vi "Main.vi"() -> ()   [LabVIEW 2018] (continued)
              tunnel: w2112 -> [w2128 w2142]
              tunnel: w2115 -> [w2127 w2155]
              tunnel: w2114 -> [w2126 w2154]
              frame False {
                n1936 = call "SQL_Update.vi"("查询语句"=w2128, "表名"="Online", "error in (no error)"=w2126, "列名对应的值"=w2135, "列名"=string[] ["Last_Station", "Last_Result", "ST403_Date", "ST403_Time", "ST403_Package_Result", "ST403_Circlip_5026621", "ST403_Jump_Ring_Data", "ST403_Jump_Ring_Tolerance", "ST402_Camera_Shield"], "connection reference"=w2127) -> ("error out"=w2130:errorcluster)  [unwired: 4 in, 1 out]
                n1937 = Unbundle By Name(w2130) -> ("status"=w2134:bool)
                n1938 = Equal?(x=w2129, y="") -> (x = y?=w2132:bool)
                n1939 = Or(x=w2134, y=w2132) -> (x .or. y?=w2131:bool)
                n1940 = case shown="假" w2131 {
                  tunnel: ["1" ("数据保存请求回复") "2" ("数据保存请求回复")] -> w2136
                  frame False {
                  }
                  frame True {
                  }
                }
              }
              frame True {
                w2150 = 0 ("索引 (行)")
                n1941 = call "SQL_Select.vi"("要读取的列名"=string[] ["[403]"], "表名"="Rework_List", "error in (no error)"=w2154, "查询语句"=w2142, "查询条件"=TRUE, "connection reference"=w2155) -> ("error out"=w2145:errorcluster, "数据"=w2151:string[][], "connection reference out"=w2146:T12)  [unwired: 3 in]
                n1942 = Index Array(array=w2151, index (row)=w2150, index (col)=w2150) -> (element=w2149:string)
                n1943 = Equal?(x=w2149, y="T") -> (x = y?=w2147:bool)
                n1944 = case shown="真" w2147 {
                  tunnel: w2146 -> [w2163 w2182]
                  tunnel: w2145 -> [w2164 w2181]
                  tunnel: w2144 -> [w2162 w2188]
                  tunnel: w2143 -> [w2159 w2183]
                  tunnel: w2142 -> [w2161 w2173]
                  tunnel: [w2158 w2175] -> w2141
                  tunnel: [w2160 w2174] -> w2140
                  frame False {
                    n1945 = call "SQL_Update.vi"("查询语句"=w2161, "表名"="Online", "error in (no error)"=w2164, "列名对应的值"=w2162, "列名"=string[] ["Last_Station", "Last_Result", "ST403_Date", "ST403_Time", "ST403_Package_Result", "ST403_Circlip_5026621", "ST403_Jump_Ring_Data", "ST403_Jump_Ring_Tolerance", "ST402_Camera_Shield"], "connection reference"=w2163) -> ("error out"=w2160:errorcluster)  [unwired: 4 in, 1 out]
                    n1946 = Unbundle By Name(w2160) -> ("status"=w2168:bool)
                    n1947 = Equal?(x=w2159, y="") -> (x = y?=w2166:bool)
                    n1948 = Or(x=w2168, y=w2166) -> (x .or. y?=w2165:bool)
                    n1949 = case shown="假" w2165 {
                      tunnel: ["1" ("数据保存请求回复") "2" ("数据保存请求回复")] -> w2158
                      frame False {
                      }
                      frame True {
                      }
                    }
                  }
                  frame True {
                    n1950 = Delete From Array(array=w2188, length=2 ("长度"), index=0 ("索引")) -> (deleted portion=w2176:string[], array with subset deleted=w2185:string[])
                    n1951 = call "SQL_Update.vi"("查询语句"=w2173, "表名"="Online", "error in (no error)"=w2181, "列名对应的值"=w2176, "列名"=string[] ["Last_Station", "Last_Result"], "connection reference"=w2182) -> ("error out"=w2180:errorcluster, "connection reference 2"=w2179:T12)  [unwired: 4 in]
                    n1952 = call "SQL_Update.vi"("查询语句"=w2173, "表名"="Rework", "error in (no error)"=w2180, "列名对应的值"=w2185, "列名"=string[] ["ST403_Date", "ST403_Time", "ST403_Package_Result", "ST403_Circlip_5026621", "ST403_Jump_Ring_Data", "ST403_Jump_Ring_Tolerance", "ST402_Camera_Shield"], "connection reference"=w2179) -> ("error out"=w2174:errorcluster)  [unwired: 4 in, 1 out]
                    n1953 = Unbundle By Name(w2174) -> ("status"=w2191:bool)
                    n1954 = Equal?(x="", y=w2183) -> (x = y?=w2190:bool)
                    n1955 = Or(x=w2191, y=w2190) -> (x .or. y?=w2189:bool)
                    n1956 = case shown="真" w2189 {
                      tunnel: ["1" ("数据保存请求回复") "2" ("数据保存请求回复")] -> w2175
                      frame False {
                      }
                      frame True {
                      }
                    }
                  }
                }
              }
            }
            n1957 = Delete From Array(array=w2088, length=2 ("长度"), index=0 ("索引")) -> (array with subset deleted=w2120:string[])  [unwired: 1 out]
            n1958 = Insert Into Array(array=string[] [] ("数组"), index=0 ("索引"), new element=w2113) -> (w2123:string[])
            n1959 = Insert Into Array(array=w2120, index=2 ("索引"), new element=w2092) -> (w2119:string[])
            n1960 = Bundle By Name(cluster=cluster{"Data":string[], "State":T1} {"Data"=[], "State"=enum."PLC通讯初始化"} ("元素"), "Data"=w2123, "State"=状态2."数据保存回复3") -> (w2122:cluster{"Data":string[], "State":T1})
            n1961 = Insert Into Array(array=string[][] [] ("数组"), index (row)=0 ("索引 (行)"), new element=w2119) -> (w2121:string[][])  [unwired: 1 in]
            n1962 = Enqueue Element(queue=w2093, element=w2122) -> ()  [unwired: 2 in, 3 out]
            n1963 = Transpose 2D Array(2D array=w2121) -> (transposed array=w2091:string[][])
            n1964 = property on="ST40-3_DATA" class="MCListbox (严格)"("ItemNames"=w2091) -> ()  [unwired: 2 in, 2 out]
            "ST403数据读取（事件）" <- FALSE ("ST403数据读取（事件）")
          }
          event "ST502扫码请求(事件)": Value Change {
            n1965 = event-data() -> ()  [unwired: 1 in, 1 out]
            n1966 = local read "502二维码"() -> (w2195:string)
            n1967 = Concatenate Strings("Where QRCode='" ("查询语句"), w2195, "'" ("字符串")) -> (w2221:string)
            n1968 = call "SQL_Select.vi"("要读取的列名"=string[] ["Last_Station", "Last_Result"], "表名"="Online", "error in (no error)"=w2200, "查询语句"=w2221, "查询条件"=TRUE, "connection reference"=w2201) -> ("error out"=w2198:errorcluster, "数据"=w2220:string[][])  [unwired: 3 in, 1 out]
            n1969 = case shown="无错误" w2198 {
              tunnel: w2220 -> [w2234 _]
              tunnel: ["1" ("右扫码请求回复") "2" ("右扫码请求回复")] -> w2213
              tunnel: [w2229 w2235] -> w2212
              tunnel: [w2228 w2235] -> w2211
              frame No Error {
                n1970 = Index Array(array=w2234, index (row)=0 ("索引 (行)")) -> (element=w2231:string[])  [unwired: 1 in]
                n1971 = Index Array(array=w2231, index #1=0 ("索引 (行)")) -> (element #1=w2229:string, element #2=w2228:string)  [unwired: 1 in]
                "上一站号 (502)" <- w2229
                "上一站结果 (502)" <- w2228
              }
              frame Error {
                w2235 = ""
              }
            }
            n1972 = Insert Into Array(array=string[] [] ("数组"), index=0 ("索引"), new element #1=w2213, new element #2=w2212, new element #3=w2211) -> (w2217:string[])
            n1973 = Format Date/Time String(time format string (%c)="%Y-%m-%d" ("时间格式字符串(%c)")) -> (date/time string=w2209:string)  [unwired: 2 in]
            n1974 = Get Date/Time String() -> (time string=w2208:string)  [unwired: 3 in, 1 out]
            n1975 = Bundle By Name(cluster=cluster{"Data":string[], "State":T1} {"Data"=[], "State"=enum."PLC通讯初始化"} ("元素"), "Data"=w2217, "State"=状态2."扫码回复") -> (w2218:cluster{"Data":string[], "State":T1})
            n1976 = Insert Into Array(array=string[] [] ("数组"), index=0 ("索引"), new element #1=w2209, new element #2=w2208, new element #3=w2195) -> (w2205:string[])
            n1977 = Enqueue Element(queue=w2199, element=w2218) -> ()  [unwired: 2 in, 3 out]
            n1978 = Insert Into Array(array=string[][] [] ("数组"), index (row)=0 ("索引 (行)"), new element=w2205) -> (w2202:string[][])  [unwired: 1 in]
            n1979 = Transpose 2D Array(2D array=w2202) -> (transposed array=w2196:string[][])
            n1980 = property on="ST50-2_DATA" class="MCListbox (严格)"("ItemNames"=w2196) -> ()  [unwired: 2 in, 2 out]
            "ST502扫码请求(事件)" <- FALSE ("ST50扫码请求(事件)")
          }
          event "ST502数据读取（事件）": Value Change {
            w2249 = 0 ("索引 (行)")
            n1981 = event-data() -> ()  [unwired: 1 in, 1 out]
            n1982 = local read "502二维码"() -> (w2237:string)
            n1983 = Dequeue Element(queue=w2260, timeout in ms (-1)=10 ("超时毫秒(-1)")) -> (element=w2241:string[])  [unwired: 1 in, 3 out]
            n1984 = Concatenate Strings("Where QRCode='" ("查询语句"), w2237, "'" ("字符串")) -> (w2251:string)
            n1985 = call "SQL_Select.vi"("要读取的列名"=string[] ["Rework_Status"], "表名"="Online", "error in (no error)"=w2243, "查询语句"=w2251, "查询条件"=TRUE, "connection reference"=w2242) -> ("error out"=w2244:errorcluster, "数据"=w2250:string[][], "connection reference out"=w2245:T12)  [unwired: 3 in]
            n1986 = Index Array(array=w2250, index (row)=w2249, index (col)=w2249) -> (element=w2248:string)
            n1987 = Equal?(x=w2248, y="T") -> (x = y?=w2246:bool)
            n1988 = case shown="真" w2246 {
              tunnel: [w2287 w2292] -> w2240
              tunnel: w2241 -> [w2286 w2295]
              tunnel: [w2281 w2291] -> w2239
              tunnel: w2237 -> [w2280 w2294]
              tunnel: w2251 -> [w2279 w2293]
              tunnel: w2245 -> [w2278 w2306]
              tunnel: w2244 -> [w2277 w2305]
              frame False {
                n1989 = call "SQL_Update.vi"("查询语句"=w2279, "表名"="Online", "error in (no error)"=w2277, "列名对应的值"=w2286, "列名"=string[] ["Last_Station", "Last_Result", "ST502_Date", "ST502_Time", "ST502_Package_Result", "ST502_Form_Seal_5026860", "ST502_Support_Ring_5027083", "ST502_O_Ring_M0104976", "ST502_Pressure_Plate_M0105053", "ST502_Camera_Shield", "ST502_Seal_Ring_TestValue", "ST502_Seal_Ring_SetValue"], "connection reference"=w2278) -> ("error out"=w2281:errorcluster)  [unwired: 4 in, 1 out]
                n1990 = Unbundle By Name(w2281) -> ("status"=w2285:bool)
                n1991 = Equal?(x=w2280, y="") -> (x = y?=w2283:bool)
                n1992 = Or(x=w2285, y=w2283) -> (x .or. y?=w2282:bool)
                n1993 = case shown="假" w2282 {
                  tunnel: ["1" ("数据保存请求回复") "2" ("数据保存请求回复")] -> w2287
                  frame False {
                  }
                  frame True {
                  }
                }
              }
              frame True {
                w2301 = 0 ("索引 (行)")
                n1994 = call "SQL_Select.vi"("要读取的列名"=string[] ["[502]"], "表名"="Rework_List", "error in (no error)"=w2305, "查询语句"=w2293, "查询条件"=TRUE, "connection reference"=w2306) -> ("error out"=w2296:errorcluster, "数据"=w2302:string[][], "connection reference out"=w2297:T12)  [unwired: 3 in]
                n1995 = Index Array(array=w2302, index (row)=w2301, index (col)=w2301) -> (element=w2300:string)
                n1996 = Equal?(x=w2300, y="T") -> (x = y?=w2298:bool)
                n1997 = case shown="假" w2298 {
                  tunnel: w2297 -> [w2314 w2333]
                  tunnel: w2296 -> [w2315 w2332]
                  tunnel: w2295 -> [w2313 w2339]
                  tunnel: w2294 -> [w2310 w2334]
                  tunnel: w2293 -> [w2312 w2324]
                  tunnel: [w2309 w2326] -> w2292
                  tunnel: [w2311 w2325] -> w2291
                  frame False {
                    n1998 = call "SQL_Update.vi"("查询语句"=w2312, "表名"="Online", "error in (no error)"=w2315, "列名对应的值"=w2313, "列名"=string[] ["Last_Station", "Last_Result", "ST502_Date", "ST502_Time", "ST502_Package_Result", "ST502_Form_Seal_5026860", "ST502_Support_Ring_5027083", "ST502_O_Ring_M0104976", "ST502_Pressure_Plate_M0105053", "ST502_Camera_Shield", "ST502_Seal_Ring_TestValue", "ST502_Seal_Ring_SetValue"], "connection reference"=w2314) -> ("error out"=w2311:errorcluster)  [unwired: 4 in, 1 out]
                    n1999 = Unbundle By Name(w2311) -> ("status"=w2319:bool)
                    n2000 = Equal?(x=w2310, y="") -> (x = y?=w2317:bool)
                    n2001 = Or(x=w2319, y=w2317) -> (x .or. y?=w2316:bool)
                    n2002 = case shown="假" w2316 {
                      tunnel: ["1" ("数据保存请求回复") "2" ("数据保存请求回复")] -> w2309
                      frame False {
                      }
                      frame True {
                      }
                    }
                  }
                  frame True {
                    n2003 = Delete From Array(array=w2339, length=2 ("长度"), index=0 ("索引")) -> (deleted portion=w2327:string[], array with subset deleted=w2336:string[])
                    n2004 = call "SQL_Update.vi"("查询语句"=w2324, "表名"="Online", "error in (no error)"=w2332, "列名对应的值"=w2327, "列名"=string[] ["Last_Station", "Last_Result"], "connection reference"=w2333) -> ("error out"=w2331:errorcluster, "connection reference 2"=w2330:T12)  [unwired: 4 in]
                    n2005 = call "SQL_Update.vi"("查询语句"=w2324, "表名"="Rework", "error in (no error)"=w2331, "列名对应的值"=w2336, "列名"=string[] ["ST502_Date", "ST502_Time", "ST502_Package_Result", "ST502_Form_Seal_5026860", "ST502_Support_Ring_5027083", "ST502_O_Ring_M0104976", "ST502_Pressure_Plate_M0105053", "ST502_Camera_Shield", "ST502_Seal_Ring_TestValue", "ST502_Seal_Ring_SetValue"], "connection reference"=w2330) -> ("error out"=w2325:errorcluster)  [unwired: 4 in, 1 out]
                    n2006 = Unbundle By Name(w2325) -> ("status"=w2342:bool)
                    n2007 = Equal?(x="", y=w2334) -> (x = y?=w2341:bool)
                    n2008 = Or(x=w2342, y=w2341) -> (x .or. y?=w2340:bool)
                    n2009 = case shown="真" w2340 {
                      tunnel: ["1" ("数据保存请求回复") "2" ("数据保存请求回复")] -> w2326
                      frame False {
                      }
                      frame True {
                      }
                    }
                  }
                }
              }
            }
            n2010 = Delete From Array(array=w2241, length=2 ("长度"), index=0 ("索引")) -> (array with subset deleted=w2263:string[])  [unwired: 1 out]
            n2011 = Insert Into Array(array=w2263, index=2 ("索引"), new element=w2237) -> (w2261:string[])
            n2012 = Insert Into Array(array=string[] [] ("数组"), index=0 ("索引"), new element=w2240) -> (w2273:string[])
            n2013 = Bundle By Name(cluster=cluster{"Data":string[], "State":T1} {"Data"=[], "State"=enum."PLC通讯初始化"} ("元素"), "Data"=w2273, "State"=状态2."数据保存回复") -> (w2269:cluster{"Data":string[], "State":T1})
            n2014 = Insert Into Array(array=string[][] [] ("数组"), index (row)=0 ("索引 (行)"), new element=w2261) -> (w2266:string[][])  [unwired: 1 in]
            n2015 = Transpose 2D Array(2D array=w2266) -> (transposed array=w2238:string[][])
            n2016 = Enqueue Element(queue=w2259, element=w2269) -> ()  [unwired: 2 in, 3 out]
            n2017 = property on="ST50-2_DATA" class="MCListbox (严格)"("ItemNames"=w2238) -> ()  [unwired: 2 in, 2 out]
            "ST502数据读取（事件）" <- FALSE ("ST50数据读取（事件）")
          }
          event "ST503扫码请求(事件)": Value Change {
            n2018 = event-data() -> ()  [unwired: 1 in, 1 out]
            n2019 = local read "503二维码"() -> (w2346:string)
            n2020 = Concatenate Strings("Where QRCode='" ("查询语句"), w2346, "'" ("字符串")) -> (w2350:string)
            n2021 = call "SQL_Select.vi"("要读取的列名"=string[] ["Last_Station", "Last_Result"], "表名"="Online", "error in (no error)"=w2348, "查询语句"=w2350, "查询条件"=TRUE, "connection reference"=w2349) -> ("error out"=w2352:errorcluster, "数据"=w2372:string[][])  [unwired: 3 in, 1 out]
            n2022 = case shown="无错误" w2352 {
              tunnel: w2372 -> [w2385 _]
              tunnel: ["1" ("右扫码请求回复") "2" ("右扫码请求回复")] -> w2365
              tunnel: [w2380 w2386] -> w2364
              tunnel: [w2379 w2386] -> w2363
              frame No Error {
                n2023 = Index Array(array=w2385, index (row)=0 ("索引 (行)")) -> (element=w2382:string[])  [unwired: 1 in]
                n2024 = Index Array(array=w2382, index #1=0 ("索引 (行)")) -> (element #1=w2380:string, element #2=w2379:string)  [unwired: 1 in]
                "上一站号 (503)" <- w2380
                "上一站结果 (503)" <- w2379
              }
              frame Error {
                w2386 = ""
              }
            }
            n2025 = Insert Into Array(array=string[] [] ("数组"), index=0 ("索引"), new element #1=w2365, new element #2=w2364, new element #3=w2363) -> (w2369:string[])
            n2026 = Format Date/Time String(time format string (%c)="%Y-%m-%d" ("时间格式字符串(%c)")) -> (date/time string=w2361:string)  [unwired: 2 in]
            n2027 = Get Date/Time String() -> (time string=w2360:string)  [unwired: 3 in, 1 out]
            n2028 = Bundle By Name(cluster=cluster{"Data":string[], "State":T1} {"Data"=[], "State"=enum."PLC通讯初始化"} ("元素"), "Data"=w2369, "State"=状态2."扫码回复2") -> (w2370:cluster{"Data":string[], "State":T1})
            n2029 = Insert Into Array(array=string[] [] ("数组"), index=0 ("索引"), new element #1=w2361, new element #2=w2360, new element #3=w2346) -> (w2357:string[])
            n2030 = Enqueue Element(queue=w2353, element=w2370) -> ()  [unwired: 2 in, 3 out]
            n2031 = Insert Into Array(array=string[][] [] ("数组"), index (row)=0 ("索引 (行)"), new element=w2357) -> (w2354:string[][])  [unwired: 1 in]
            n2032 = Transpose 2D Array(2D array=w2354) -> (transposed array=w2347:string[][])
            n2033 = property on="ST50-3_DATA" class="MCListbox (严格)"("ItemNames"=w2347) -> ()  [unwired: 2 in, 2 out]
            "ST503扫码请求(事件)" <- FALSE ("ST502扫码请求(事件)")
          }
          event "ST503数据读取（事件）": Value Change {
            w2405 = 0 ("索引 (行)")
            n2034 = event-data() -> ()  [unwired: 1 in, 1 out]
            n2035 = local read "503二维码"() -> (w2396:string)
            n2036 = Concatenate Strings("Where QRCode='" ("查询语句"), w2396, "'" ("字符串")) -> (w2397:string)
            n2037 = call "SQL_Select.vi"("要读取的列名"=string[] ["Rework_Status"], "表名"="Online", "error in (no error)"=w2394, "查询语句"=w2397, "查询条件"=TRUE, "connection reference"=w2395) -> ("error out"=w2400:errorcluster, "数据"=w2406:string[][], "connection reference out"=w2401:T12)  [unwired: 3 in]
            n2038 = local read "503读取数据"() -> (w2388:string[])
            n2039 = Index Array(array=w2406, index (row)=w2405, index (col)=w2405) -> (element=w2404:string)
            n2040 = Equal?(x=w2404, y="T") -> (x = y?=w2402:bool)
            n2041 = case shown="真" w2402 {
              tunnel: [w2436 w2441] -> w2399
              tunnel: w2388 -> [w2435 w2444]
              tunnel: [w2430 w2440] -> w2398
              tunnel: w2396 -> [w2429 w2443]
              tunnel: w2397 -> [w2428 w2442]
              tunnel: w2401 -> [w2427 w2455]
              tunnel: w2400 -> [w2426 w2454]
              frame False {
                n2042 = call "SQL_Update.vi"("查询语句"=w2428, "表名"="Online", "error in (no error)"=w2426, "列名对应的值"=w2435, "列名"=string[] ["Last_Station", "Last_Result", "ST503_Date", "ST503_Time", "ST503_Package_Result"], "connection reference"=w2427) -> ("error out"=w2430:errorcluster)  [unwired: 4 in, 1 out]
                n2043 = Unbundle By Name(w2430) -> ("status"=w2434:bool)
                n2044 = Equal?(x=w2429, y="") -> (x = y?=w2432:bool)
                n2045 = Or(x=w2434, y=w2432) -> (x .or. y?=w2431:bool)
                n2046 = case shown="假" w2431 {
                  tunnel: ["1" ("数据保存请求回复") "2" ("数据保存请求回复")] -> w2436
                  frame False {
                  }
                  frame True {
                  }
                }
              }
              frame True {
                w2450 = 0 ("索引 (行)")
                n2047 = call "SQL_Select.vi"("要读取的列名"=string[] ["[503]"], "表名"="Rework_List", "error in (no error)"=w2454, "查询语句"=w2442, "查询条件"=TRUE, "connection reference"=w2455) -> ("error out"=w2445:errorcluster, "数据"=w2451:string[][], "connection reference out"=w2446:T12)  [unwired: 3 in]
                n2048 = Index Array(array=w2451, index (row)=w2450, index (col)=w2450) -> (element=w2449:string)
                n2049 = Equal?(x=w2449, y="T") -> (x = y?=w2447:bool)
                n2050 = case shown="真" w2447 {
                  tunnel: w2446 -> [w2463 w2482]
                  tunnel: w2445 -> [w2464 w2481]
                  tunnel: w2444 -> [w2462 w2488]
                  tunnel: w2443 -> [w2459 w2483]
                  tunnel: w2442 -> [w2461 w2473]
                  tunnel: [w2458 w2475] -> w2441
                  tunnel: [w2460 w2474] -> w2440
                  frame False {
                    n2051 = call "SQL_Update.vi"("查询语句"=w2461, "表名"="Online", "error in (no error)"=w2464, "列名对应的值"=w2462, "列名"=string[] ["Last_Station", "Last_Result", "ST503_Date", "ST503_Time", "ST503_Package_Result"], "connection reference"=w2463) -> ("error out"=w2460:errorcluster)  [unwired: 4 in, 1 out]
                    n2052 = Unbundle By Name(w2460) -> ("status"=w2468:bool)
                    n2053 = Equal?(x=w2459, y="") -> (x = y?=w2466:bool)
                    n2054 = Or(x=w2468, y=w2466) -> (x .or. y?=w2465:bool)
                    n2055 = case shown="假" w2465 {
                      tunnel: ["1" ("数据保存请求回复") "2" ("数据保存请求回复")] -> w2458
                      frame False {
                      }
                      frame True {
                      }
                    }
                  }
                  frame True {
                    n2056 = Delete From Array(array=w2488, length=2 ("长度"), index=0 ("索引")) -> (deleted portion=w2476:string[], array with subset deleted=w2485:string[])
                    n2057 = call "SQL_Update.vi"("查询语句"=w2473, "表名"="Online", "error in (no error)"=w2481, "列名对应的值"=w2476, "列名"=string[] ["Last_Station", "Last_Result"], "connection reference"=w2482) -> ("error out"=w2480:errorcluster, "connection reference 2"=w2479:T12)  [unwired: 4 in]
                    n2058 = call "SQL_Update.vi"("查询语句"=w2473, "表名"="Rework", "error in (no error)"=w2480, "列名对应的值"=w2485, "列名"=string[] ["ST503_Date", "ST503_Time", "ST503_Package_Result"], "connection reference"=w2479) -> ("error out"=w2474:errorcluster)  [unwired: 4 in, 1 out]
                    n2059 = Unbundle By Name(w2474) -> ("status"=w2491:bool)
                    n2060 = Equal?(x="", y=w2483) -> (x = y?=w2490:bool)
                    n2061 = Or(x=w2491, y=w2490) -> (x .or. y?=w2489:bool)
                    n2062 = case shown="真" w2489 {
                      tunnel: ["1" ("数据保存请求回复") "2" ("数据保存请求回复")] -> w2475
                      frame False {
                      }
                      frame True {
                      }
                    }
                  }
                }
              }
            }
            n2063 = Delete From Array(array=w2388, length=2 ("长度"), index=0 ("索引")) -> (array with subset deleted=w2415:string[])  [unwired: 1 out]
            n2064 = Insert Into Array(array=string[] [] ("数组"), index=0 ("索引"), new element=w2399) -> (w2422:string[])
            n2065 = Insert Into Array(array=w2415, index=2 ("索引"), new element=w2396) -> (w2391:string[])
            n2066 = Bundle By Name(cluster=cluster{"Data":string[], "State":T1} {"Data"=[], "State"=enum."PLC通讯初始化"} ("元素"), "Data"=w2422, "State"=状态2."数据保存回复2") -> (w2418:cluster{"Data":string[], "State":T1})
            n2067 = Insert Into Array(array=string[][] [] ("数组"), index (row)=0 ("索引 (行)"), new element=w2391) -> (w2390:string[][])  [unwired: 1 in]
            n2068 = Enqueue Element(queue=w2413, element=w2418) -> ()  [unwired: 2 in, 3 out]
            n2069 = Transpose 2D Array(2D array=w2390) -> (transposed array=w2389:string[][])
            n2070 = property on="ST50-3_DATA" class="MCListbox (严格)"("ItemNames"=w2389) -> ()  [unwired: 2 in, 2 out]
            "ST503数据读取（事件）" <- FALSE ("ST502数据读取（事件）")
          }
          event "ST601扫码请求(事件)": Value Change {
            n2071 = event-data() -> ()  [unwired: 1 in, 1 out]
            n2072 = local read "601二维码"() -> (w2495:string)
            n2073 = Concatenate Strings("Where QRCode='" ("查询语句"), w2495, "'" ("字符串")) -> (w2521:string)
            n2074 = call "SQL_Select.vi"("要读取的列名"=string[] ["Last_Station", "Last_Result"], "表名"="Online", "error in (no error)"=w2500, "查询语句"=w2521, "查询条件"=TRUE, "connection reference"=w2501) -> ("error out"=w2498:errorcluster, "数据"=w2520:string[][])  [unwired: 3 in, 1 out]
            n2075 = case shown="无错误" w2498 {
              tunnel: w2520 -> [w2534 _]
              tunnel: ["1" ("右扫码请求回复") "2" ("右扫码请求回复")] -> w2513
              tunnel: [w2529 w2535] -> w2512
              tunnel: [w2528 w2535] -> w2511
              frame No Error {
                n2076 = Index Array(array=w2534, index (row)=0 ("索引 (行)")) -> (element=w2531:string[])  [unwired: 1 in]
                n2077 = Index Array(array=w2531, index #1=0 ("索引 (行)")) -> (element #1=w2529:string, element #2=w2528:string)  [unwired: 1 in]
                "上一站号 (601)" <- w2529
                "上一站结果 (601)" <- w2528
              }
              frame Error {
                w2535 = ""
              }
            }
            n2078 = Insert Into Array(array=string[] [] ("数组"), index=0 ("索引"), new element #1=w2513, new element #2=w2512, new element #3=w2511) -> (w2517:string[])
            n2079 = Format Date/Time String(time format string (%c)="%Y-%m-%d" ("时间格式字符串(%c)")) -> (date/time string=w2509:string)  [unwired: 2 in]
            n2080 = Get Date/Time String() -> (time string=w2508:string)  [unwired: 3 in, 1 out]
            n2081 = Bundle By Name(cluster=cluster{"Data":string[], "State":T1} {"Data"=[], "State"=enum."PLC通讯初始化"} ("元素"), "Data"=w2517, "State"=状态2."扫码回复") -> (w2518:cluster{"Data":string[], "State":T1})
            n2082 = Insert Into Array(array=string[] [] ("数组"), index=0 ("索引"), new element #1=w2509, new element #2=w2508, new element #3=w2495) -> (w2505:string[])
            n2083 = Enqueue Element(queue=w2499, element=w2518) -> ()  [unwired: 2 in, 3 out]
            n2084 = Insert Into Array(array=string[][] [] ("数组"), index (row)=0 ("索引 (行)"), new element=w2505) -> (w2502:string[][])  [unwired: 1 in]
            n2085 = Transpose 2D Array(2D array=w2502) -> (transposed array=w2496:string[][])
            n2086 = property on="ST60-1_DATA" class="MCListbox (严格)"("ItemNames"=w2496) -> ()  [unwired: 2 in, 2 out]
            "ST601扫码请求(事件)" <- FALSE ("ST60扫码请求(事件)")
          }
          event "ST601数据读取（事件）": Value Change {
            w2551 = 0 ("索引 (行)")
            n2087 = event-data() -> ()  [unwired: 1 in, 1 out]
            n2088 = Dequeue Element(queue=w2540, timeout in ms (-1)=10 ("超时毫秒(-1)")) -> (element=w2539:string[])  [unwired: 1 in, 3 out]
            n2089 = local read "601二维码"() -> (w2538:string)
            n2090 = Concatenate Strings("Where QRCode='" ("查询语句"), w2538, "'" ("字符串")) -> (w2553:string)
            n2091 = call "SQL_Select.vi"("要读取的列名"=string[] ["Rework_Status"], "表名"="Online", "error in (no error)"=w2545, "查询语句"=w2553, "查询条件"=TRUE, "connection reference"=w2544) -> ("error out"=w2546:errorcluster, "数据"=w2552:string[][], "connection reference out"=w2547:T12)  [unwired: 3 in]
            n2092 = Index Array(array=w2552, index (row)=w2551, index (col)=w2551) -> (element=w2550:string)
            n2093 = Equal?(x=w2550, y="T") -> (x = y?=w2548:bool)
            n2094 = case shown="假" w2548 {
              tunnel: [w2587 w2592] -> w2542
              tunnel: w2539 -> [w2586 w2595]
              tunnel: [w2581 w2591] -> w2543
              tunnel: w2538 -> [w2580 w2594]
              tunnel: w2553 -> [w2579 w2593]
              tunnel: w2547 -> [w2578 w2606]
              tunnel: w2546 -> [w2577 w2605]
              frame False {
                n2095 = call "SQL_Update.vi"("查询语句"=w2579, "表名"="Online", "error in (no error)"=w2577, "列名对应的值"=w2586, "列名"=string[] ["Last_Station", "Last_Result", "ST601_Date", "ST601_Time", "ST601_Package_Result", "ST601_Disk_Spring_5024300", "ST601_Sleeve_5020302", "ST601_Eclip_5018568"], "connection reference"=w2578) -> ("error out"=w2581:errorcluster)  [unwired: 4 in, 1 out]
                n2096 = Unbundle By Name(w2581) -> ("status"=w2585:bool)
                n2097 = Equal?(x=w2580, y="") -> (x = y?=w2583:bool)
                n2098 = Or(x=w2585, y=w2583) -> (x .or. y?=w2582:bool)
                n2099 = case shown="假" w2582 {
                  tunnel: ["1" ("数据保存请求回复") "2" ("数据保存请求回复")] -> w2587
                  frame False {
                  }
                  frame True {
                  }
                }
              }
              frame True {
                w2601 = 0 ("索引 (行)")
                n2100 = call "SQL_Select.vi"("要读取的列名"=string[] ["[601]"], "表名"="Rework_List", "error in (no error)"=w2605, "查询语句"=w2593, "查询条件"=TRUE, "connection reference"=w2606) -> ("error out"=w2596:errorcluster, "数据"=w2602:string[][], "connection reference out"=w2597:T12)  [unwired: 3 in]
                n2101 = Index Array(array=w2602, index (row)=w2601, index (col)=w2601) -> (element=w2600:string)
                n2102 = Equal?(x=w2600, y="T") -> (x = y?=w2598:bool)
                n2103 = case shown="真" w2598 {
                  tunnel: w2597 -> [w2614 w2633]
                  tunnel: w2596 -> [w2615 w2632]
                  tunnel: w2595 -> [w2613 w2639]
                  tunnel: w2594 -> [w2610 w2634]
                  tunnel: w2593 -> [w2612 w2624]
                  tunnel: [w2609 w2626] -> w2592
                  tunnel: [w2611 w2625] -> w2591
                  frame False {
                    n2104 = call "SQL_Update.vi"("查询语句"=w2612, "表名"="Online", "error in (no error)"=w2615, "列名对应的值"=w2613, "列名"=string[] ["Last_Station", "Last_Result", "ST601_Date", "ST601_Time", "ST601_Package_Result", "ST601_Disk_Spring_5024300", "ST601_Sleeve_5020302", "ST601_Eclip_5018568"], "connection reference"=w2614) -> ("error out"=w2611:errorcluster)  [unwired: 4 in, 1 out]
                    n2105 = Unbundle By Name(w2611) -> ("status"=w2619:bool)
                    n2106 = Equal?(x=w2610, y="") -> (x = y?=w2617:bool)
                    n2107 = Or(x=w2619, y=w2617) -> (x .or. y?=w2616:bool)
                    n2108 = case shown="假" w2616 {
                      tunnel: ["1" ("数据保存请求回复") "2" ("数据保存请求回复")] -> w2609
                      frame False {
                      }
                      frame True {
                      }
                    }
                  }
                  frame True {
                    n2109 = Delete From Array(array=w2639, length=2 ("长度"), index=0 ("索引")) -> (deleted portion=w2627:string[], array with subset deleted=w2636:string[])
                    n2110 = call "SQL_Update.vi"("查询语句"=w2624, "表名"="Online", "error in (no error)"=w2632, "列名对应的值"=w2627, "列名"=string[] ["Last_Station", "Last_Result"], "connection reference"=w2633) -> ("error out"=w2631:errorcluster, "connection reference 2"=w2630:T12)  [unwired: 4 in]
                    n2111 = call "SQL_Update.vi"("查询语句"=w2624, "表名"="Rework", "error in (no error)"=w2631, "列名对应的值"=w2636, "列名"=string[] ["ST601_Date", "ST601_Time", "ST601_Package_Result", "ST601_Disk_Spring_5024300", "ST601_Sleeve_5020302", "ST601_Eclip_5018568"], "connection reference"=w2630) -> ("error out"=w2625:errorcluster)  [unwired: 4 in, 1 out]
                    n2112 = Unbundle By Name(w2625) -> ("status"=w2642:bool)
                    n2113 = Equal?(x="", y=w2634) -> (x = y?=w2641:bool)
                    n2114 = Or(x=w2642, y=w2641) -> (x .or. y?=w2640:bool)
                    n2115 = case shown="真" w2640 {
                      tunnel: ["1" ("数据保存请求回复") "2" ("数据保存请求回复")] -> w2626
                      frame False {
                      }
                      frame True {
                      }
                    }
                  }
                }
              }
            }
            n2116 = Delete From Array(array=w2539, length=2 ("长度"), index=0 ("索引")) -> (array with subset deleted=w2563:string[])  [unwired: 1 out]
            n2117 = Insert Into Array(array=string[] [] ("数组"), index=0 ("索引"), new element=w2542) -> (w2573:string[])
            n2118 = Bundle By Name(cluster=cluster{"Data":string[], "State":T1} {"Data"=[], "State"=enum."PLC通讯初始化"} ("元素"), "Data"=w2573, "State"=状态2."数据保存回复") -> (w2569:cluster{"Data":string[], "State":T1})
            n2119 = Insert Into Array(array=w2563, index=2 ("索引"), new element=w2538) -> (w2561:string[])
            n2120 = Enqueue Element(queue=w2560, element=w2569) -> ()  [unwired: 2 in, 3 out]
            n2121 = Insert Into Array(array=string[][] [] ("数组"), index (row)=0 ("索引 (行)"), new element=w2561) -> (w2566:string[][])  [unwired: 1 in]
            n2122 = Transpose 2D Array(2D array=w2566) -> (transposed array=w2537:string[][])
            n2123 = property on="ST60-1_DATA" class="MCListbox (严格)"("ItemNames"=w2537) -> ()  [unwired: 2 in, 2 out]
            "ST601数据读取（事件）" <- FALSE ("ST60数据读取（事件）")
          }
          event "ST602扫码请求(事件)": Value Change {
            n2124 = event-data() -> ()  [unwired: 1 in, 2 out]
            n2125 = local read "602二维码"() -> (w2646:string)
            n2126 = Concatenate Strings("Where QRCode='" ("查询语句"), w2646, "'" ("字符串")) -> (w2672:string)
            n2127 = call "SQL_Select.vi"("要读取的列名"=string[] ["Last_Station", "Last_Result"], "表名"="Online", "error in (no error)"=w2652, "查询语句"=w2672, "查询条件"=TRUE, "connection reference"=w2651) -> ("error out"=w2650:errorcluster, "数据"=w2671:string[][])  [unwired: 3 in, 1 out]
            n2128 = case shown="无错误" w2650 {
              tunnel: w2671 -> [w2685 _]
              tunnel: ["1" ("右扫码请求回复") "2" ("右扫码请求回复")] -> w2664
              tunnel: [w2680 w2686] -> w2663
              tunnel: [w2679 w2686] -> w2662
              frame No Error {
                n2129 = Index Array(array=w2685, index (row)=0 ("索引 (行)")) -> (element=w2682:string[])  [unwired: 1 in]
                n2130 = Index Array(array=w2682, index #1=0 ("索引 (行)")) -> (element #1=w2680:string, element #2=w2679:string)  [unwired: 1 in]
                "上一站号 (602)" <- w2680
                "上一站结果 (602)" <- w2679
              }
              frame Error {
                w2686 = ""
              }
            }
            n2131 = Insert Into Array(array=string[] [] ("数组"), index=0 ("索引"), new element #1=w2664, new element #2=w2663, new element #3=w2662) -> (w2668:string[])
            n2132 = Format Date/Time String(time format string (%c)="%Y-%m-%d" ("时间格式字符串(%c)")) -> (date/time string=w2660:string)  [unwired: 2 in]
            n2133 = Get Date/Time String() -> (time string=w2659:string)  [unwired: 3 in, 1 out]
            n2134 = Bundle By Name(cluster=cluster{"Data":string[], "State":T1} {"Data"=[], "State"=enum."PLC通讯初始化"} ("元素"), "Data"=w2668, "State"=状态2."扫码回复2") -> (w2669:cluster{"Data":string[], "State":T1})
            n2135 = Insert Into Array(array=string[] [] ("数组"), index=0 ("索引"), new element #1=w2660, new element #2=w2659, new element #3=w2646) -> (w2656:string[])
            n2136 = Enqueue Element(queue=w2647, element=w2669) -> ()  [unwired: 2 in, 3 out]
            n2137 = Insert Into Array(array=string[][] [] ("数组"), index (row)=0 ("索引 (行)"), new element=w2656) -> (w2653:string[][])  [unwired: 1 in]
            n2138 = Transpose 2D Array(2D array=w2653) -> (transposed array=w2648:string[][])
            n2139 = property on="ST60-2_DATA" class="MCListbox (严格)"("ItemNames"=w2648) -> ()  [unwired: 2 in, 2 out]
            "ST602扫码请求(事件)" <- FALSE ("ST702扫码请求(事件)")
          }
          event "ST602数据读取(事件)": Value Change {
            w2702 = 0 ("索引 (行)")
            n2140 = event-data() -> ()  [unwired: 1 in, 2 out]
            n2141 = local read "602二维码"() -> (w2692:string)
            n2142 = Concatenate Strings("Where QRCode='" ("查询语句"), w2692, "'" ("字符串")) -> (w2704:string)
            n2143 = local read "602读取数据"() -> (w2688:string[])
            n2144 = call "SQL_Select.vi"("要读取的列名"=string[] ["Rework_Status"], "表名"="Online", "error in (no error)"=w2695, "查询语句"=w2704, "查询条件"=TRUE, "connection reference"=w2696) -> ("error out"=w2697:errorcluster, "数据"=w2703:string[][], "connection reference out"=w2698:T12)  [unwired: 3 in]
            n2145 = Index Array(array=w2703, index (row)=w2702, index (col)=w2702) -> (element=w2701:string)
            n2146 = Equal?(x=w2701, y="T") -> (x = y?=w2699:bool)
            n2147 = case shown="真" w2699 {
              tunnel: [w2736 w2741] -> w2693
              tunnel: w2688 -> [w2735 w2744]
              tunnel: [w2730 w2740] -> w2694
              tunnel: w2692 -> [w2729 w2743]
              tunnel: w2704 -> [w2728 w2742]
              tunnel: w2698 -> [w2727 w2755]
              tunnel: w2697 -> [w2726 w2754]
              frame False {
                n2148 = call "SQL_Update.vi"("查询语句"=w2728, "表名"="Online", "error in (no error)"=w2726, "列名对应的值"=w2735, "列名"=string[] ["Last_Station", "Last_Result", "ST602_Date", "ST602_Time", "ST602_Package_Result"], "connection reference"=w2727) -> ("error out"=w2730:errorcluster)  [unwired: 4 in, 1 out]
                n2149 = Unbundle By Name(w2730) -> ("status"=w2734:bool)
                n2150 = Equal?(x=w2729, y="") -> (x = y?=w2732:bool)
                n2151 = Or(x=w2734, y=w2732) -> (x .or. y?=w2731:bool)
                n2152 = case shown="假" w2731 {
                  tunnel: ["1" ("数据保存请求回复") "2" ("数据保存请求回复")] -> w2736
                  frame False {
                  }
                  frame True {
                  }
                }
              }
              frame True {
                w2750 = 0 ("索引 (行)")
                n2153 = call "SQL_Select.vi"("要读取的列名"=string[] ["[602]"], "表名"="Rework_List", "error in (no error)"=w2754, "查询语句"=w2742, "查询条件"=TRUE, "connection reference"=w2755) -> ("error out"=w2745:errorcluster, "数据"=w2751:string[][], "connection reference out"=w2746:T12)  [unwired: 3 in]
                n2154 = Index Array(array=w2751, index (row)=w2750, index (col)=w2750) -> (element=w2749:string)
                n2155 = Equal?(x=w2749, y="T") -> (x = y?=w2747:bool)
                n2156 = case shown="真" w2747 {
                  tunnel: w2746 -> [w2763 w2782]
                  tunnel: w2745 -> [w2764 w2781]
                  tunnel: w2744 -> [w2762 w2788]
                  tunnel: w2743 -> [w2759 w2783]
                  tunnel: w2742 -> [w2761 w2773]
                  tunnel: [w2758 w2775] -> w2741
                  tunnel: [w2760 w2774] -> w2740
                  frame False {
                    n2157 = call "SQL_Update.vi"("查询语句"=w2761, "表名"="Online", "error in (no error)"=w2764, "列名对应的值"=w2762, "列名"=string[] ["Last_Station", "Last_Result", "ST602_Date", "ST602_Time", "ST602_Package_Result"], "connection reference"=w2763) -> ("error out"=w2760:errorcluster)  [unwired: 4 in, 1 out]
                    n2158 = Unbundle By Name(w2760) -> ("status"=w2768:bool)
                    n2159 = Equal?(x=w2759, y="") -> (x = y?=w2766:bool)
                    n2160 = Or(x=w2768, y=w2766) -> (x .or. y?=w2765:bool)
                    n2161 = case shown="假" w2765 {
                      tunnel: ["1" ("数据保存请求回复") "2" ("数据保存请求回复")] -> w2758
                      frame False {
                      }
                      frame True {
                      }
                    }
                  }
                  frame True {
                    n2162 = Delete From Array(array=w2788, length=2 ("长度"), index=0 ("索引")) -> (deleted portion=w2776:string[], array with subset deleted=w2785:string[])
                    n2163 = call "SQL_Update.vi"("查询语句"=w2773, "表名"="Online", "error in (no error)"=w2781, "列名对应的值"=w2776, "列名"=string[] ["Last_Station", "Last_Result"], "connection reference"=w2782) -> ("error out"=w2780:errorcluster, "connection reference 2"=w2779:T12)  [unwired: 4 in]
                    n2164 = call "SQL_Update.vi"("查询语句"=w2773, "表名"="Rework", "error in (no error)"=w2780, "列名对应的值"=w2785, "列名"=string[] ["ST602_Date", "ST602_Time", "ST602_Package_Result"], "connection reference"=w2779) -> ("error out"=w2774:errorcluster)  [unwired: 4 in, 1 out]
                    n2165 = Unbundle By Name(w2774) -> ("status"=w2791:bool)
                    n2166 = Equal?(x="", y=w2783) -> (x = y?=w2790:bool)
                    n2167 = Or(x=w2791, y=w2790) -> (x .or. y?=w2789:bool)
                    n2168 = case shown="真" w2789 {
                      tunnel: ["1" ("数据保存请求回复") "2" ("数据保存请求回复")] -> w2775
                      frame False {
                      }
                      frame True {
                      }
                    }
                  }
                }
              }
            }
            n2169 = Delete From Array(array=w2688, length=2 ("长度"), index=0 ("索引")) -> (array with subset deleted=w2712:string[])  [unwired: 1 out]
            n2170 = Insert Into Array(array=string[] [] ("数组"), index=0 ("索引"), new element=w2693) -> (w2722:string[])
            n2171 = Insert Into Array(array=w2712, index=2 ("索引"), new element=w2692) -> (w2691:string[])
            n2172 = Bundle By Name(cluster=cluster{"Data":string[], "State":T1} {"Data"=[], "State"=enum."PLC通讯初始化"} ("元素"), "Data"=w2722, "State"=状态2."数据保存回复2") -> (w2718:cluster{"Data":string[], "State":T1})
            n2173 = Enqueue Element(queue=w2689, element=w2718) -> ()  [unwired: 2 in, 3 out]
            n2174 = Insert Into Array(array=string[][] [] ("数组"), index (row)=0 ("索引 (行)"), new element=w2691) -> (w2715:string[][])  [unwired: 1 in]
            n2175 = Transpose 2D Array(2D array=w2715) -> (transposed array=w2690:string[][])
            n2176 = property on="ST60-2_DATA" class="MCListbox (严格)"("ItemNames"=w2690) -> ()  [unwired: 2 in, 2 out]
            "ST602数据读取(事件)" <- FALSE ("ST702数据读取(事件)")
          }
          event "ST802扫码请求(事件)": Value Change {
            n2177 = event-data() -> ()  [unwired: 1 in, 1 out]
            n2178 = local read "802二维码"() -> (w2798:string)
            n2179 = Concatenate Strings("Where QRCode='" ("查询语句"), w2798, "'" ("字符串")) -> (w2796:string)
            n2180 = call "SQL_Select.vi"("要读取的列名"=string[] ["Last_Station", "Last_Result"], "表名"="Online", "error in (no error)"=w2801, "查询语句"=w2796, "查询条件"=TRUE, "connection reference"=w2802) -> ("error out"=w2800:errorcluster, "数据"=w2812:string[][])  [unwired: 3 in, 1 out]
            n2181 = local write "802查询条件"(w2796) -> ()
            n2182 = case shown="无错误" w2800 {
              tunnel: w2812 -> [w2824 _]
              tunnel: ["1" ("右扫码请求回复") "2" ("右扫码请求回复")] -> w2805
              tunnel: [w2819 w2825] -> w2804
              tunnel: [w2818 w2825] -> w2803
              frame No Error {
                n2183 = Index Array(array=w2824, index (row)=0 ("索引 (行)")) -> (element=w2821:string[])  [unwired: 1 in]
                n2184 = Index Array(array=w2821, index #1=0 ("索引 (行)")) -> (element #1=w2819:string, element #2=w2818:string)  [unwired: 1 in]
                "上一站号 (802)" <- w2819
                "上一站结果 (802)" <- w2818
              }
              frame Error {
                w2825 = ""
              }
            }
            n2185 = Insert Into Array(array=string[] [] ("数组"), index=0 ("索引"), new element #1=w2805, new element #2=w2804, new element #3=w2803) -> (w2809:string[])
            n2186 = Bundle By Name(cluster=cluster{"Data":string[], "State":T1} {"Data"=[], "State"=enum."PLC通讯初始化"} ("元素"), "Data"=w2809, "State"=状态2."扫码回复2") -> (w2810:cluster{"Data":string[], "State":T1})
            n2187 = Enqueue Element(queue=w2797, element=w2810) -> ()  [unwired: 2 in, 3 out]
            "ST802扫码请求(事件)" <- FALSE ("ST70扫码请求(事件)")
          }
          event "ST802保存数据(事件)": Value Change {
            w2862 = 0 ("索引 (行)")
            n2188 = event-data() -> ()  [unwired: 1 in, 1 out]
            n2189 = local read "802二维码"() -> (w2837:string)
            n2190 = Concatenate Strings("Where QRCode='" ("查询语句"), w2837, "'" ("字符串")) -> (w2843:string)
            n2191 = local read "802数据"() -> (w2852:string[])
            n2192 = call "SQL_Select.vi"("要读取的列名"=string[] ["Rework_Status"], "表名"="Online", "error in (no error)"=w2855, "查询语句"=w2843, "查询条件"=TRUE, "connection reference"=w2856) -> ("error out"=w2857:errorcluster, "数据"=w2863:string[][], "connection reference out"=w2858:T12)  [unwired: 3 in]
            n2193 = Index Array(array=w2863, index (row)=w2862, index (col)=w2862) -> (element=w2861:string)
            n2194 = Equal?(x=w2861, y="T") -> (x = y?=w2859:bool)
            n2195 = case shown="假" w2859 {
              tunnel: [w2912 w2918] -> w2854
              tunnel: w2852 -> [w2911 w2921]
              tunnel: [w2906 w2917] -> w2848
              tunnel: w2837 -> [w2905 w2920]
              tunnel: w2843 -> [w2901 w2919]
              tunnel: w2858 -> [w2904 w2932]
              tunnel: w2857 -> [w2903 w2931]
              tunnel: [w2900 w2916] -> w2851
              frame False {
                n2196 = call "SQL_Update.vi"("查询语句"=w2901, "表名"="Online", "error in (no error)"=w2903, "列名对应的值"=w2911, "列名"=string[] ["Last_Station", "Last_Result", "ST80_Date", "ST80_Time", "Marking_Code", "ST80_Marking_Code_Class"], "connection reference"=w2904) -> ("error out"=w2906:errorcluster, "connection reference 2"=w2900:T12)  [unwired: 4 in]
                n2197 = Unbundle By Name(w2906) -> ("status"=w2910:bool)
                n2198 = Equal?(x=w2905, y="") -> (x = y?=w2908:bool)
                n2199 = Or(x=w2910, y=w2908) -> (x .or. y?=w2907:bool)
                n2200 = case shown="假" w2907 {
                  tunnel: ["1" ("数据保存请求回复") "2" ("数据保存请求回复")] -> w2912
                  frame False {
                  }
                  frame True {
                  }
                }
              }
              frame True {
                w2927 = 0 ("索引 (行)")
                n2201 = call "SQL_Select.vi"("要读取的列名"=string[] ["[80]"], "表名"="Rework_List", "error in (no error)"=w2931, "查询语句"=w2919, "查询条件"=TRUE, "connection reference"=w2932) -> ("error out"=w2922:errorcluster, "数据"=w2928:string[][], "connection reference out"=w2923:T12)  [unwired: 3 in]
                n2202 = Index Array(array=w2928, index (row)=w2927, index (col)=w2927) -> (element=w2926:string)
                n2203 = Equal?(x=w2926, y="T") -> (x = y?=w2924:bool)
                n2204 = case shown="真" w2924 {
                  tunnel: w2923 -> [w2941 w2961]
                  tunnel: w2922 -> [w2942 w2960]
                  tunnel: w2921 -> [w2940 w2967]
                  tunnel: w2920 -> [w2937 w2962]
                  tunnel: w2919 -> [w2939 w2952]
                  tunnel: [w2936 w2954] -> w2918
                  tunnel: [w2938 w2953] -> w2917
                  tunnel: [w2934 w2950] -> w2916
                  frame False {
                    n2205 = call "SQL_Update.vi"("查询语句"=w2939, "表名"="Online", "error in (no error)"=w2942, "列名对应的值"=w2940, "列名"=string[] ["Last_Station", "Last_Result", "ST80_Date", "ST80_Time", "Marking_Code", "ST80_Marking_Code_Class"], "connection reference"=w2941) -> ("error out"=w2938:errorcluster, "connection reference 2"=w2934:T12)  [unwired: 4 in]
                    n2206 = Unbundle By Name(w2938) -> ("status"=w2946:bool)
                    n2207 = Equal?(x=w2937, y="") -> (x = y?=w2944:bool)
                    n2208 = Or(x=w2946, y=w2944) -> (x .or. y?=w2943:bool)
                    n2209 = case shown="假" w2943 {
                      tunnel: ["1" ("数据保存请求回复") "2" ("数据保存请求回复")] -> w2936
                      frame False {
                      }
                      frame True {
                      }
                    }
                  }
                  frame True {
                    n2210 = Delete From Array(array=w2967, length=2 ("长度"), index=0 ("索引")) -> (deleted portion=w2955:string[], array with subset deleted=w2964:string[])
                    n2211 = call "SQL_Update.vi"("查询语句"=w2952, "表名"="Online", "error in (no error)"=w2960, "列名对应的值"=w2955, "列名"=string[] ["Last_Station", "Last_Result"], "connection reference"=w2961) -> ("error out"=w2959:errorcluster, "connection reference 2"=w2958:T12)  [unwired: 4 in]
                    n2212 = call "SQL_Update.vi"("查询语句"=w2952, "表名"="Rework", "error in (no error)"=w2959, "列名对应的值"=w2964, "列名"=string[] ["ST80_Date", "ST80_Time", "Marking_Code", "ST80_Marking_Code_Class"], "connection reference"=w2958) -> ("error out"=w2953:errorcluster, "connection reference 2"=w2950:T12)  [unwired: 4 in]
                    n2213 = Unbundle By Name(w2953) -> ("status"=w2970:bool)
                    n2214 = Equal?(x="", y=w2962) -> (x = y?=w2969:bool)
                    n2215 = Or(x=w2970, y=w2969) -> (x .or. y?=w2968:bool)
                    n2216 = case shown="假" w2968 {
                      tunnel: ["1" ("数据保存请求回复") "2" ("数据保存请求回复")] -> w2954
                      frame False {
                      }
                      frame True {
                      }
                    }
                  }
                }
              }
            }
            n2217 = Insert Into Array(array=string[] [] ("数组"), index=0 ("索引"), new element=w2854) -> (w2873:string[])
            n2218 = call "SQL_Select.vi"("表名"="Online", "error in (no error)"=w2848, "查询语句"=w2843, "查询条件"=TRUE, "connection reference"=w2851) -> ("error out"=w2846:errorcluster, "数据"=w2845:string[][], "connection reference out"=w2847:T12)  [unwired: 4 in]
            n2219 = Bundle By Name(cluster=cluster{"Data":string[], "State":T1} {"Data"=[], "State"=enum."PLC通讯初始化"} ("元素"), "Data"=w2873, "State"=状态2."数据保存回复2") -> (w2869:cluster{"Data":string[], "State":T1})
            n2220 = Index Array(array=w2845, index (row)=0 ("索引 (行)")) -> (element=w2832:string[])  [unwired: 1 in]
            n2221 = Enqueue Element(queue=w2853, element=w2869) -> ()  [unwired: 2 in, 3 out]
            n2222 = Index Array(array=w2832, index #1=7 ("索引")) -> (element #1=w2830:string, element #2=w2829:string)  [unwired: 1 in]
            n2223 = Equal?(x=w2830, y="80") -> (x = y?=w2833:bool)
            n2224 = Equal?(x=w2829, y="OK") -> (x = y?=w2834:bool)
            n2225 = And(x=w2833, y=w2834) -> (x .and. y?=w2828:bool)
            n2226 = case shown="假" w2828 {
              tunnel: w2847 -> [_ w2885]
              tunnel: w2846 -> [w2875 w2884]
              tunnel: w2832 -> [_ w2883]
              tunnel: [w2875 w2882] -> w2841
              tunnel: w2837 -> [_ w2881]
              frame False {
              }
              frame True {
                n2227 = call <vilib>:"DB Tools List Columns.vi"("error in (no error)"=w2884, "table"="Offline" ("表名"), "connection reference"=w2885) -> ("error out"=w2897:errorcluster, "columns"=w2898:string[], "connection reference out"=w2899:T12)  [unwired: 1 in, 1 out]
                n2228 = Delete From Array(array=w2883, length=1 ("长度"), index=0 ("索引")) -> (array with subset deleted=w2880:string[])  [unwired: 1 out]
                n2229 = Format Date/Time String(time format string (%c)="%Y-%m-%d_%H:%M" ("时间格式字符串(%c)")) -> (date/time string=w2877:string)  [unwired: 2 in]
                n2230 = Delete From Array(array=w2898, length=1 ("长度"), index=0 ("索引")) -> (array with subset deleted=w2896:string[])  [unwired: 1 out]
                n2231 = Replace Array Subset(array=w2880, new element=w2877, index=3 ("索引")) -> (w2876:string[])
                n2232 = call "SQL_Insert.vi"("表名"="Offline", "error in (no error)"=w2897, "值"=w2876, "列名"=w2896, "connection reference"=w2899) -> ("error out"=w2894:errorcluster, "connection reference 2"=w2895:T12)  [unwired: 5 in]
                n2233 = call "SQL_Delete.vi"("表名"="Online", "error in (no error)"=w2894, "值"=w2881, "列名"="QRCode", "connection reference"=w2895) -> ("error out"=w2882:errorcluster)  [unwired: 5 in, 1 out]
              }
            }
            n2234 = Unbundle By Name(w2841) -> ("source"=w2839:string)
            n2235 = Concatenate Strings("ST802 数据保存错误  ", w2837, " " ("字符串"), w2839) -> (w2840:string)
            "ST802保存数据(事件)" <- FALSE ("ST70数据读取(事件)")
          }
          event "ST80扫码请求(事件)": Value Change {
            w2981 = "Online" ("表名")
            n2236 = event-data() -> ()  [unwired: 1 in, 2 out]
            n2237 = local read "80二维码"() -> (w2982:string)
            n2238 = Concatenate Strings(" Where QRCode='" ("查询语句"), w2982, "'" ("字符串")) -> (w2974:string)
            "802查询条件" <- w2974
            n2239 = call "SQL_Select.vi"("表名"=w2981, "error in (no error)"=w2975, "查询语句"=w2974, "查询条件"=TRUE, "connection reference"=w2980) -> ("error out"=w2977:errorcluster, "数据"=w2978:string[][], "connection reference out"=w2979:T12)  [unwired: 4 in]
            n2240 = Matrix Size(0:w2978) -> (1:w2990:i32)  [unwired: 1 out]
            n2241 = Equal To 0?(x=w2990) -> (x = 0?=w2991:bool)
            n2242 = case shown="假" w2991 {
              tunnel: w2987 -> [w3000 w3056]
              tunnel: w2977 -> [w2999 w3069]
              tunnel: w2979 -> [w2996 w3071]
              tunnel: w2981 -> [_ _]
              tunnel: w2978 -> [w2997 _]
              tunnel: w2982 -> [w2994 _]
              tunnel: [w2993 w3055] -> w2986
              tunnel: w2974 -> [_ w3070]
              frame False {
                n2243 = Index Array(array=w2997, index (row)=0 ("索引 (行)")) -> (element=w2995:string[])  [unwired: 1 in]
                n2244 = case shown="无错误" w2999 {
                  selector: w2999 -> [_ w3050]
                  tunnel: ["1" ("右扫码请求回复") "2" ("右扫码请求回复")] -> w3003
                  tunnel: [w3012 w3051] -> w3002
                  tunnel: [w3019 w3051] -> w3001
                  tunnel: w2995 -> [w3021 _]
                  tunnel: w2996 -> [w3015 _]
                  tunnel: w2995 -> [w3014 _]
                  tunnel: w2994 -> [w3010 _]
                  tunnel: [w3013 w3050] -> w2993
                  frame No Error {
                    n2245 = Index Array(array=w3021, index #1=7 ("索引 (行)")) -> (element #1=w3012:string, element #2=w3019:string)  [unwired: 1 in]
                    "上一站号 (80)" <- w3012
                    "上一站结果 (80)" <- w3019
                    n2246 = Equal?(x=w3012, y="70") -> (x = y?=w3011:bool)
                    n2247 = Equal?(x=w3019, y="OK") -> (x = y?=w3017:bool)
                    n2248 = And(x=w3011, y=w3017) -> (x .and. y?=w3016:bool)
                    n2249 = case shown="真" w3016 {
                      tunnel: w3015 -> [_ w3030]
                      tunnel: w3014 -> [_ w3029]
                      tunnel: w3010 -> [_ w3027]
                      tunnel: [errorcluster {"status"=FALSE, "code"=0, "source"=""} ("error out") w3028] -> w3013
                      frame False {
                      }
                      frame True {
                        n2250 = Format Date/Time String(time format string (%c)="%Y-%m-%d_%H:%M" ("时间格式字符串(%c)")) -> (date/time string=w3042:string)  [unwired: 2 in]
                        n2251 = call <vilib>:"DB Tools List Columns.vi"("table"="Offline" ("表名"), "connection reference"=w3030) -> ("error out"=w3047:errorcluster, "columns"=w3048:string[], "connection reference out"=w3049:T12)  [unwired: 2 in, 1 out]
                        n2252 = Delete From Array(array=w3029, length=1 ("长度"), index=0 ("索引")) -> (array with subset deleted=w3043:string[])  [unwired: 1 out]
                        n2253 = Delete From Array(array=w3048, length=1 ("长度"), index=0 ("索引")) -> (array with subset deleted=w3046:string[])  [unwired: 1 out]
                        n2254 = Replace Array Subset(array=w3043, new element #1=w3042, index #1=3 ("索引"), new element #2="80" ("新元素/子数组"), index #2=6 ("索引")) -> (w3041:string[])
                        n2255 = call "SQL_Insert.vi"("表名"="Offline", "error in (no error)"=w3047, "值"=w3041, "列名"=w3046, "connection reference"=w3049) -> ("error out"=w3044:errorcluster, "connection reference 2"=w3045:T12)  [unwired: 5 in]
                        n2256 = call "SQL_Delete.vi"("表名"="Online", "error in (no error)"=w3044, "值"=w3027, "列名"="QRCode", "connection reference"=w3045) -> ("error out"=w3028:errorcluster)  [unwired: 5 in, 1 out]
                      }
                    }
                  }
                  frame Error {
                    w3051 = ""
                  }
                }
                n2257 = Insert Into Array(array=string[] [] ("数组"), index=0 ("索引"), new element #1=w3003, new element #2=w3002, new element #3=w3001) -> (w3007:string[])
                n2258 = Bundle By Name(cluster=cluster{"Data":string[], "State":T1} {"Data"=[], "State"=enum."PLC通讯初始化"} ("元素"), "Data"=w3007, "State"=状态2."扫码回复") -> (w3008:cluster{"Data":string[], "State":T1})
                n2259 = Enqueue Element(queue=w3000, element=w3008) -> ()  [unwired: 2 in, 3 out]
              }
              frame True {
                n2260 = call "SQL_Select.vi"("要读取的列名"=string[] ["Last_Station", "Last_Result"], "表名"="Offline", "error in (no error)"=w3069, "查询语句"=w3070, "查询条件"=TRUE, "connection reference"=w3071) -> ("error out"=w3055:errorcluster, "数据"=w3057:string[][])  [unwired: 3 in, 1 out]
                n2261 = Index Array(array=w3057, index (row)=0 ("索引 (行)")) -> (element=w3058:string[])  [unwired: 1 in]
                n2262 = case shown="错误" w3055 {
                  tunnel: ["1" ("右扫码请求回复") "2" ("右扫码请求回复")] -> w3062
                  tunnel: [w3074 w3078] -> w3061
                  tunnel: [w3073 w3078] -> w3060
                  tunnel: w3058 -> [w3075 _]
                  frame No Error {
                    n2263 = Index Array(array=w3075, index #1=0 ("索引 (行)")) -> (element #1=w3074:string, element #2=w3073:string)  [unwired: 1 in]
                    n2264 = local write "上一站号 (80)"(w3074) -> ()
                    n2265 = local write "上一站结果 (80)"(w3073) -> ()
                  }
                  frame Error {
                    w3078 = ""
                  }
                }
